vi "I64.vi"(4 "Value":i64) -> (1 "Constant":refnum<class "Abs_I64 Integer.lvclass">)   [LabVIEW 2021, in "Const_I64.lvclass"]
uses:
  Const_I64.lvclass
  Abs_Types/I64 Integer/Abs_I64 Integer.lvclass
  C:/Program Files (x86)/National Instruments/LabVIEW 2021/vi.lib/TSA/Abstract Data Classes/Abs_Types/I64 Integer/Abs_I64 Integer.lvclass
  Const_I64.lvclass/Const_I64.ctl
  Properties/Write Value.vi
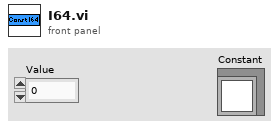
[diagram p1: front panel]
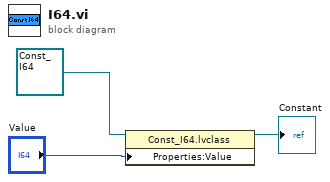
[diagram p0: block diagram]
diagram:
  n1 = property class="Const_I64.lvclass"(reference=refnum<class "Const_I64.lvclass"> refnum ("Constants.lvlib:Numeric.lvclass"), "Properties:Value"="Value") -> (reference out=→"Constant":refnum<class "Const_I64.lvclass">)  [unwired: 1 in, 1 out]
